vi "Overlay VI.vi"(2 "error in (no error)":errorcluster, 3 "Object coordinates":T1, 4 "Input text":string, 5 "Input image":T2) -> (0 "error out":errorcluster, 1 "Image":T2(plugin-control))   [LabVIEW 2018]
uses:
  <vilib>/vision/Image Controls.llb/IMAQ Image.ctl
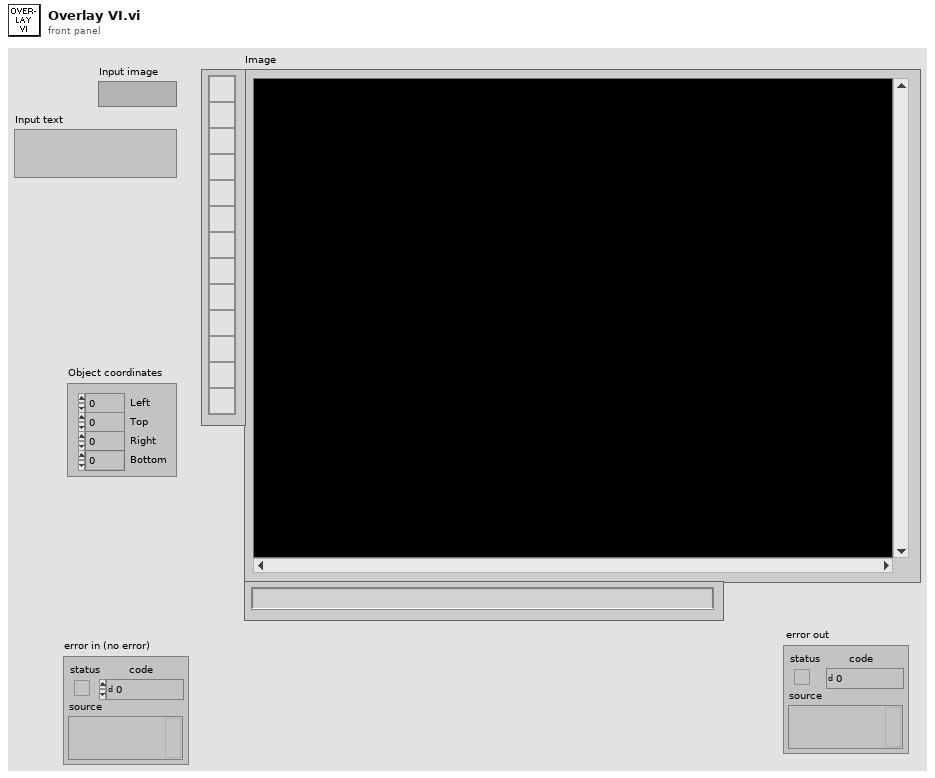
[diagram p1: front panel]
types:
  T1 = cluster{"Left":i32, "Top":i32, "Right":i32, "Bottom":i32}
  T2 = typedef "IMAQ Image.ctl" = refnum<image>
  T3 = cluster{"Desired Font (Application)":enum16{"User-specified Font", "Application Font", "System Font", "Dialog Font"}, "[User-specified Font]":cluster{"Font Name":string, "Size":i16, "Strikeout?":bool, "Italic?":bool, "Underline?":bool, "Outline?":bool, "Shadow?":bool, "Bold?":bool, "Rotation Angle":dbl}, "Horizontal Alignment":i16, "Vertical Alignment":i16}
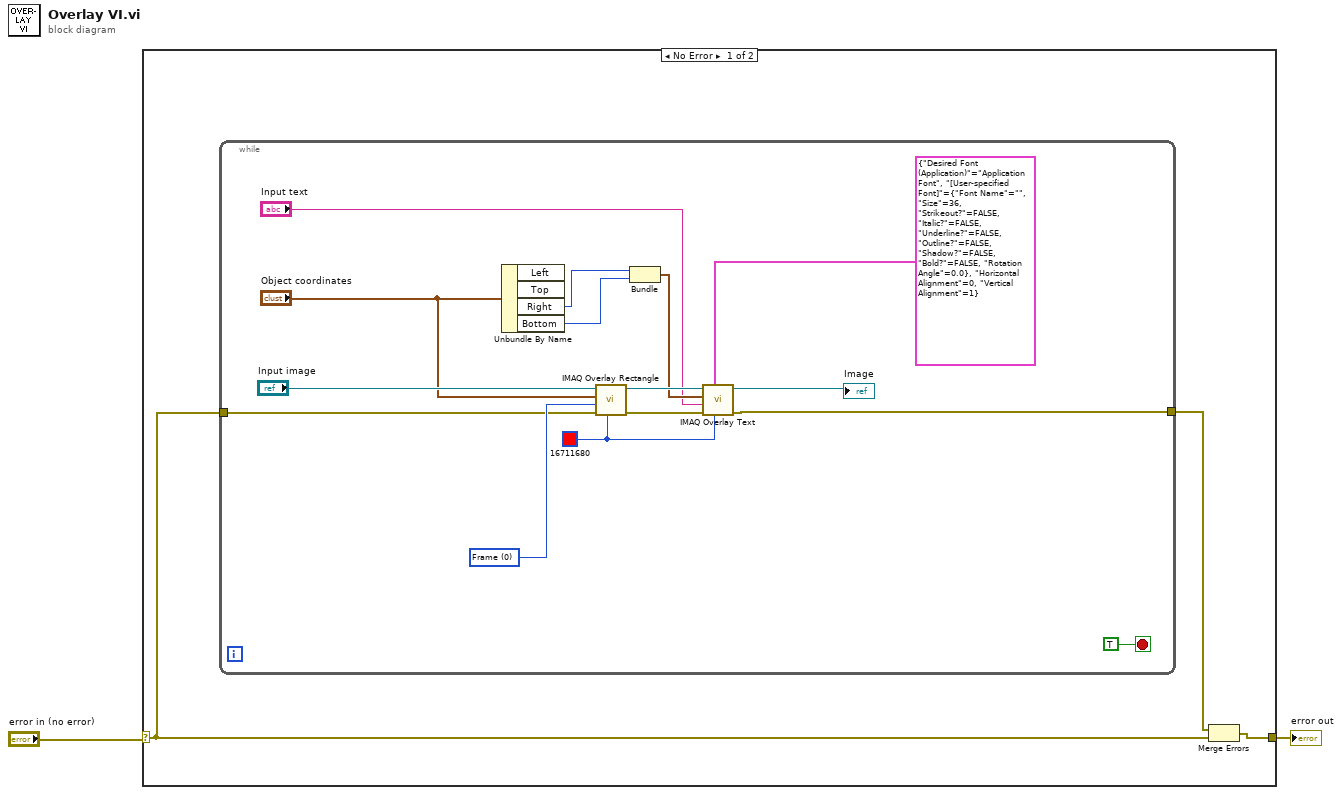
[diagram p0: block diagram]
diagram:
  n1 = case shown="No Error" "error in (no error)" {
    selector: "error in (no error)" -> [w5 w21]
    tunnel: [w3 w21] -> w1
    frame No Error {
      n2 = while {
        tunnel: w5 -> [w19]
        tunnel: [w15] -> w4
        stop <- TRUE stop-if-true
        w9 = u32 16711680 ("Color")
        w20 = u32 0 items=["Frame", "Fill", "Highlight"] ("Drawing Mode (Frame)")
        n3 = Unbundle By Name("Object coordinates") -> ("Right"=w7:i32, "Bottom"=w6:i32)  [unwired: 2 out]
        n4 = call "IMAQ Overlay Rectangle"("Color"=w9, "error in (no error)"=w19, "Drawing Mode (Frame)"=w20, "Rectangle"="Object coordinates", "Image"="Input image") -> ("error out"=w16:errorcluster, "Image Out"=w17:T2)  [unwired: 5 in]
        n5 = Bundle("Right"=w7, "Bottom"=w6) -> (w11:cluster{"Right":i32, "Bottom":i32})  [unwired: 1 in]
        n6 = call "IMAQ Overlay Text"("Text Color (black)"=w9, "Font, Size & Style"=T3 {"Desired Font (Application)"=enum."Application Font", "[User-specified Font]"={"Font Name"="", "Size"=36, "Strikeout?"=FALSE, "Italic?"=FALSE, "Underline?"=FALSE, "Outline?"=FALSE, "Shadow?"=FALSE, "Bold?"=FALSE, "Rotation Angle"=0.0}, "Horizontal Alignment"=0, "Vertical Alignment"=1}, "error in (no error)"=w16, "String"="Input text", "Origin"=w11, "Image"=w17) -> ("error out"=w15:errorcluster, "Image Out"=→"Image":T2)  [unwired: 4 in]
      }
      n7 = Merge Errors(w4, w5) -> (w3:errorcluster)
    }
    frame Error {
    }
  }
  "error out" <- w1
